vi "2_Trav_move.vi"(1 "Extra Command String":string, 3 "Home Z":T1, 5 "New Position":sgl[](array[numeric])=[0.0, 0.0, 0.0] format="%.2f", 9 "Backlash Compensation?":bool=TRUE, 11 "Simulate/Run":T2, 12 "Row Number":i32=-1, 13 "Currently on Point":i32=-1, 14 "Last Part of Move?":bool=TRUE) -> (4 "Trav Position achieved":sgl[](array[numeric]) format="%.2f", 6 "Error from Traverse named":string, 15 "Error String":string)   [LabVIEW 2022 SP3]
uses:
  Controls/User_Specific_mode.ctl
  Controls/Home.ctl
  Controls/Tunnel_Coordinates.ctl
  Globals/Extra_Commands_Global.vi
  Globals/Trav_pos_global.vi
  Globals/Constants_global.vi
panel:
  out "Offset (Tun Cord) 1-2":sgl[](array[numeric])
  out "Steps for 1st Traverse":sgl[][](array[numeric])
  out "File Content":string[](array[string])
  out "Traverse files":path[](array[path])
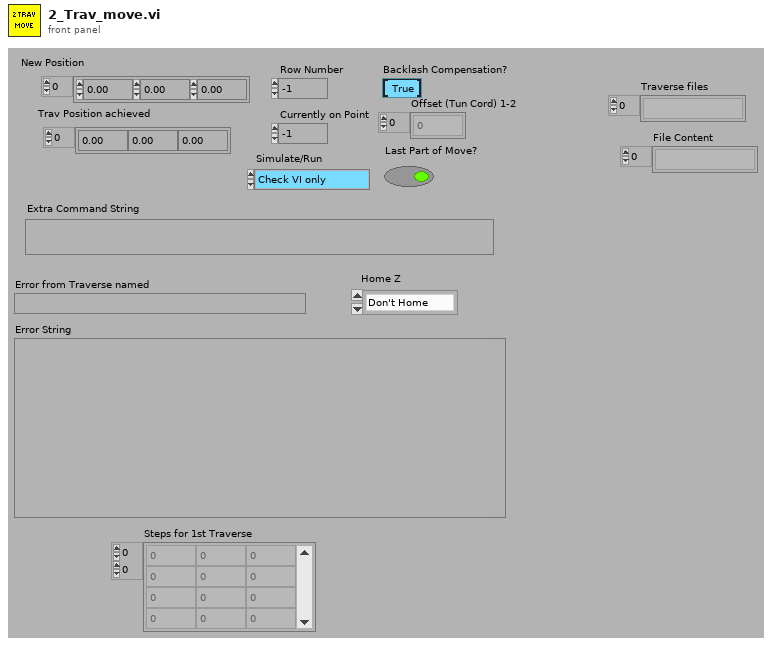
[diagram p1: front panel]
types:
  T1 = typedef "Home.ctl" = enum16{"Don't Home", "Home  +X", "Home  -X", "Home  +Y", "Home  -Y", "Home  +Z", "Home  -Z"}
  T2 = typedef "User_Specific_mode.ctl" = enum16{"Check VI only", "Run VI"}
  T3 = typedef "Tunnel_Coordinates.ctl" = enum16{"Work in Tunnel Coordinates", "Work in Model Coordinates"}
  T4 = enum16{"To Traverse Coordinates", "To User Coordinates"}
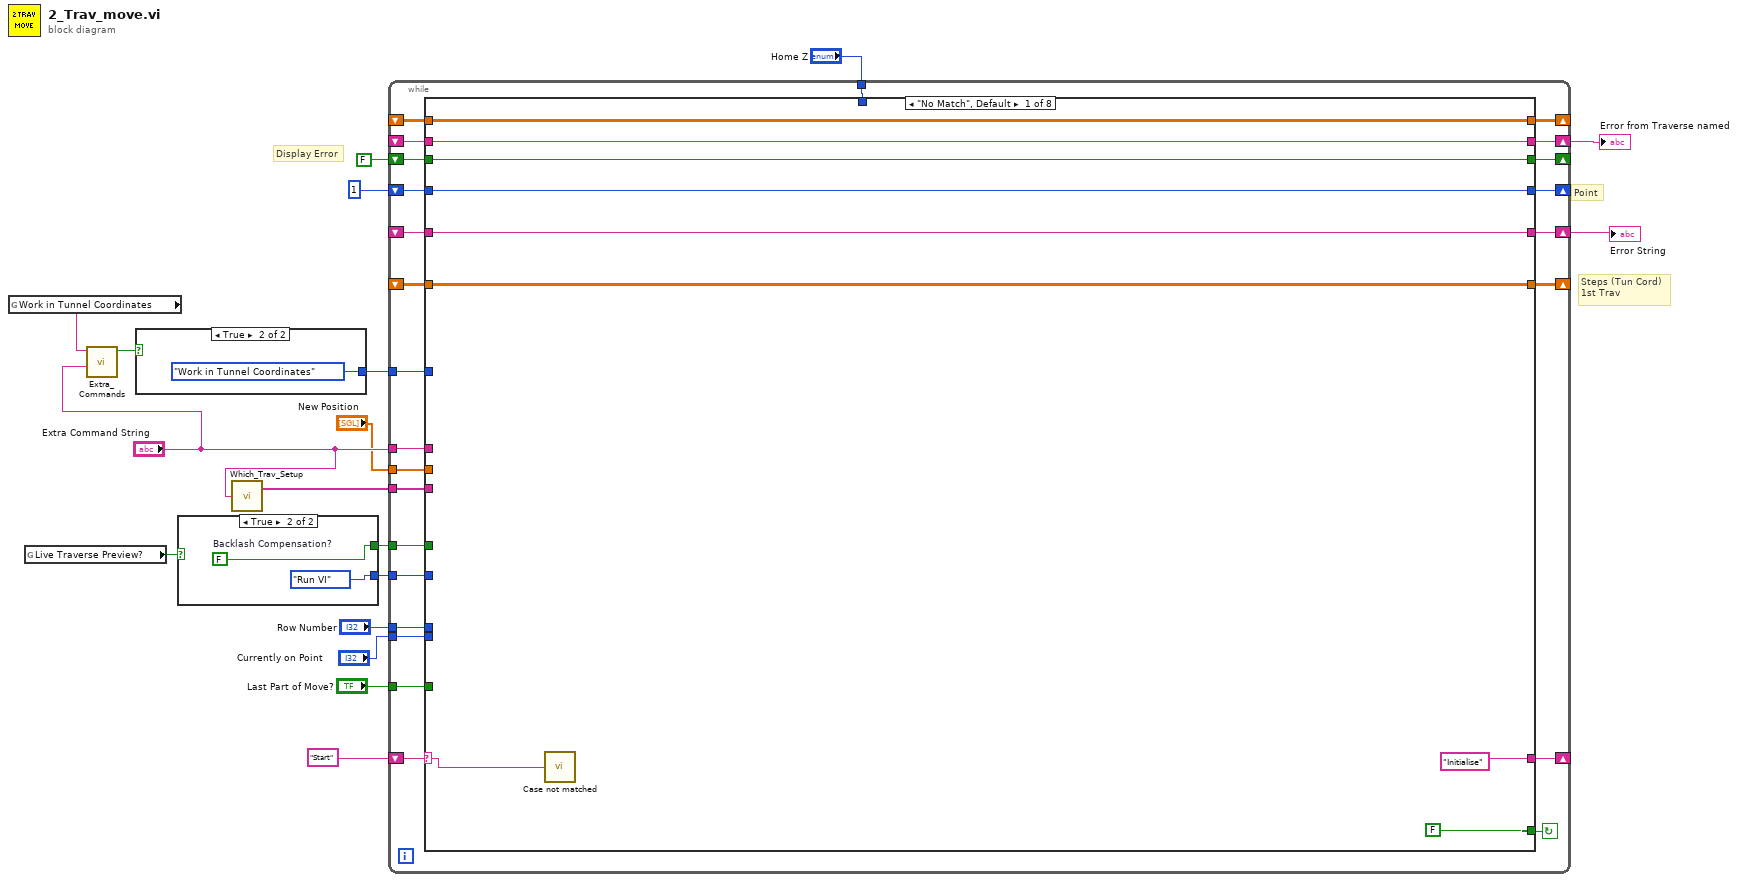
[diagram p0: block diagram]
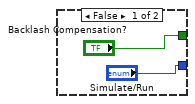
[diagram p2: hidden frame]
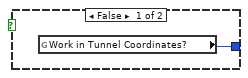
[diagram p3: hidden frame]
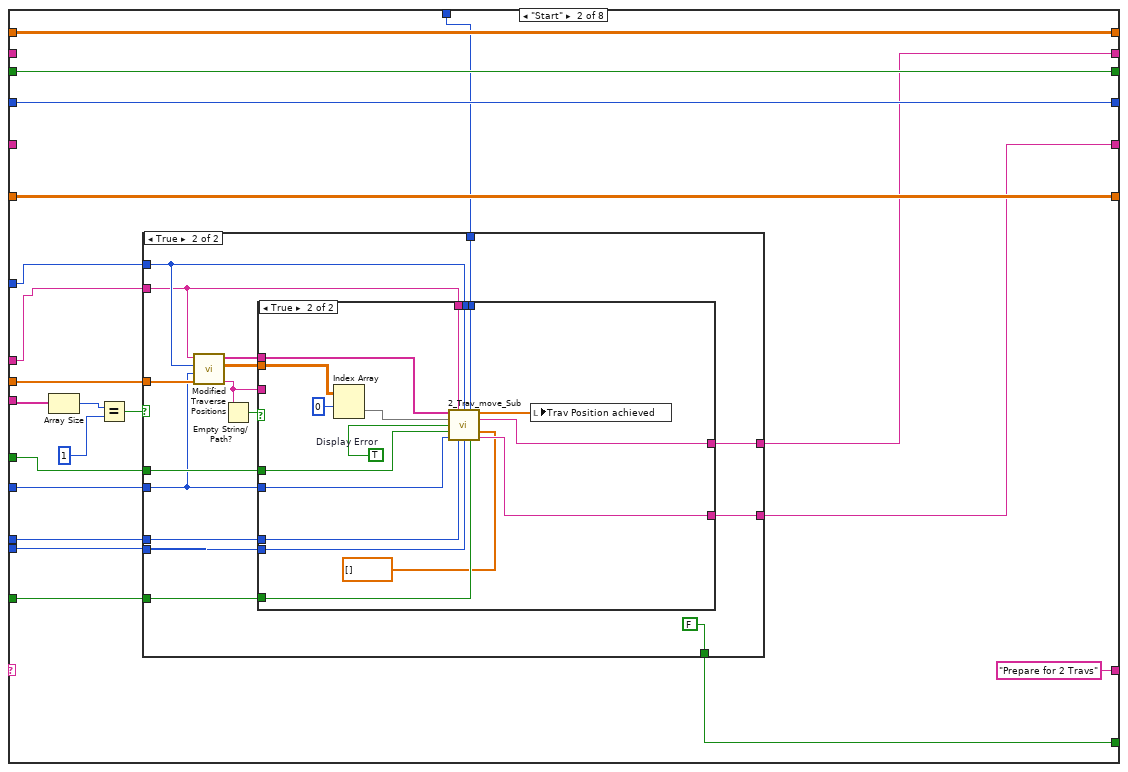
[diagram p4: hidden frame]
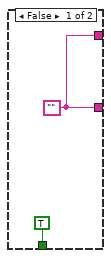
[diagram p5: hidden frame]
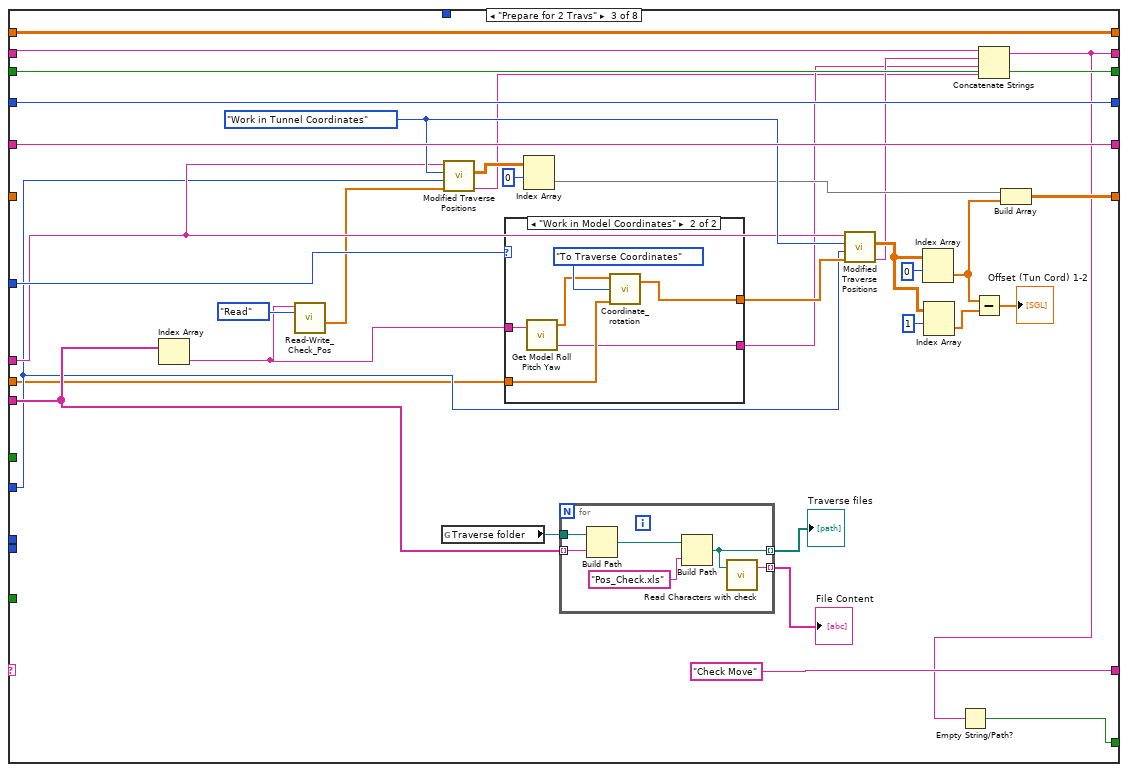
[diagram p7: hidden frame]
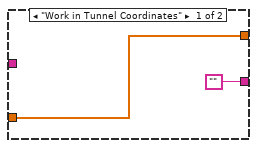
[diagram p8: hidden frame]
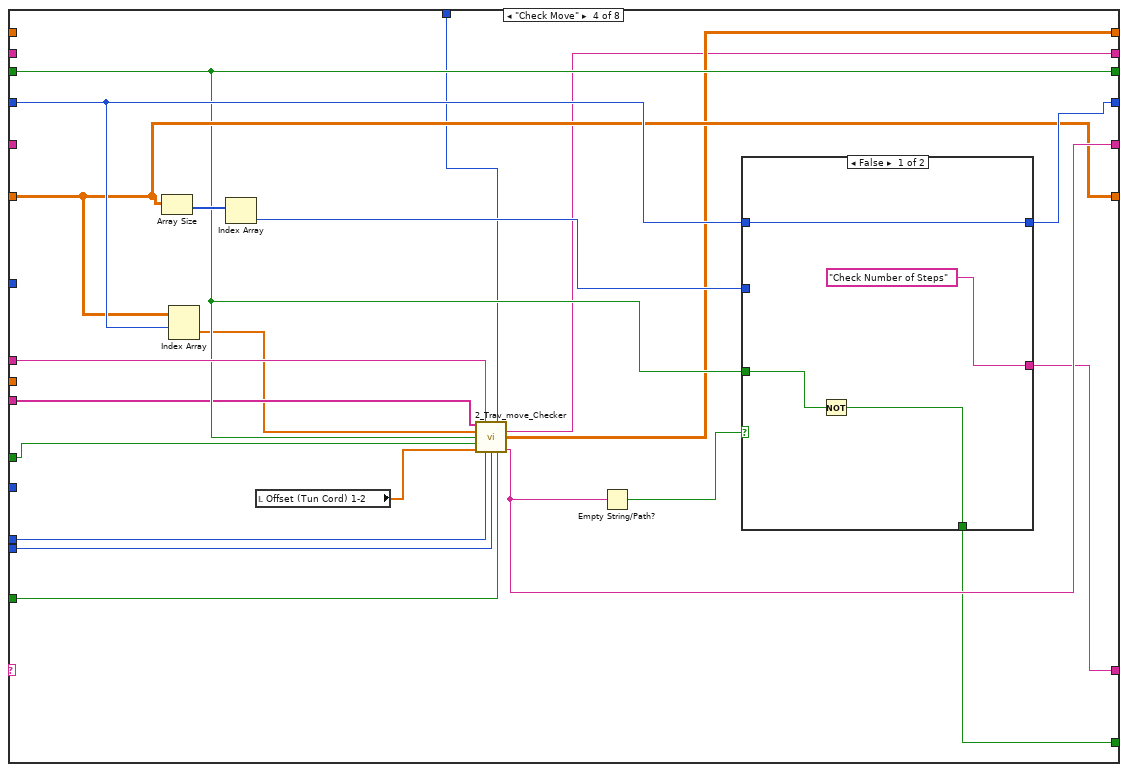
[diagram p9: hidden frame]
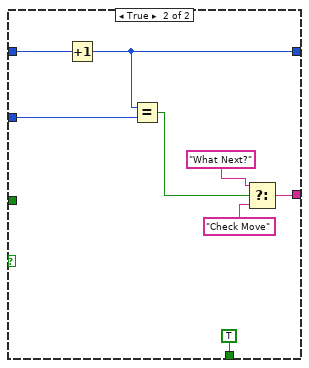
[diagram p10: hidden frame]
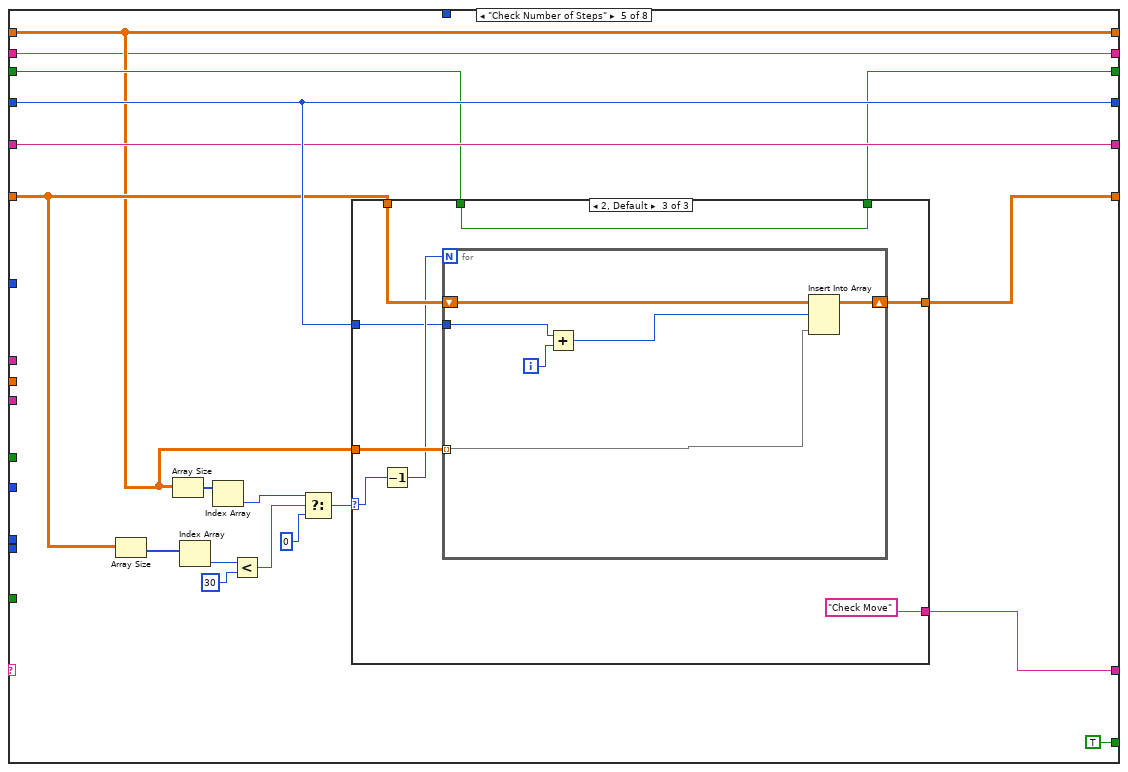
[diagram p11: hidden frame]
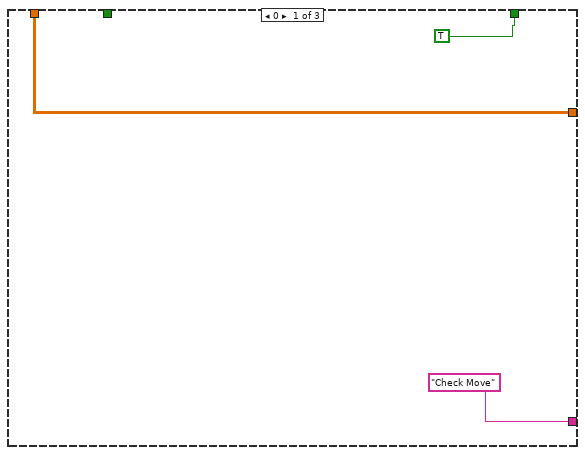
[diagram p12: hidden frame]
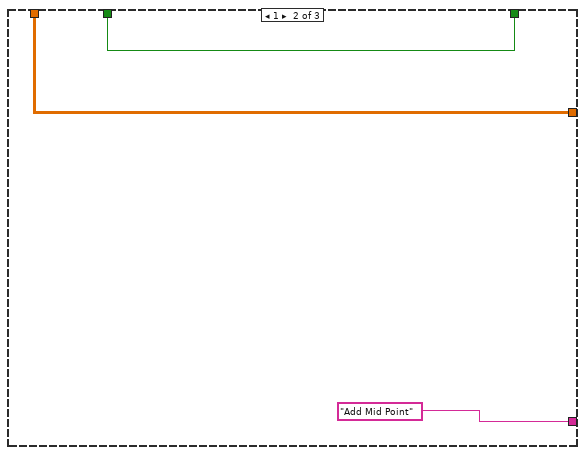
[diagram p13: hidden frame]
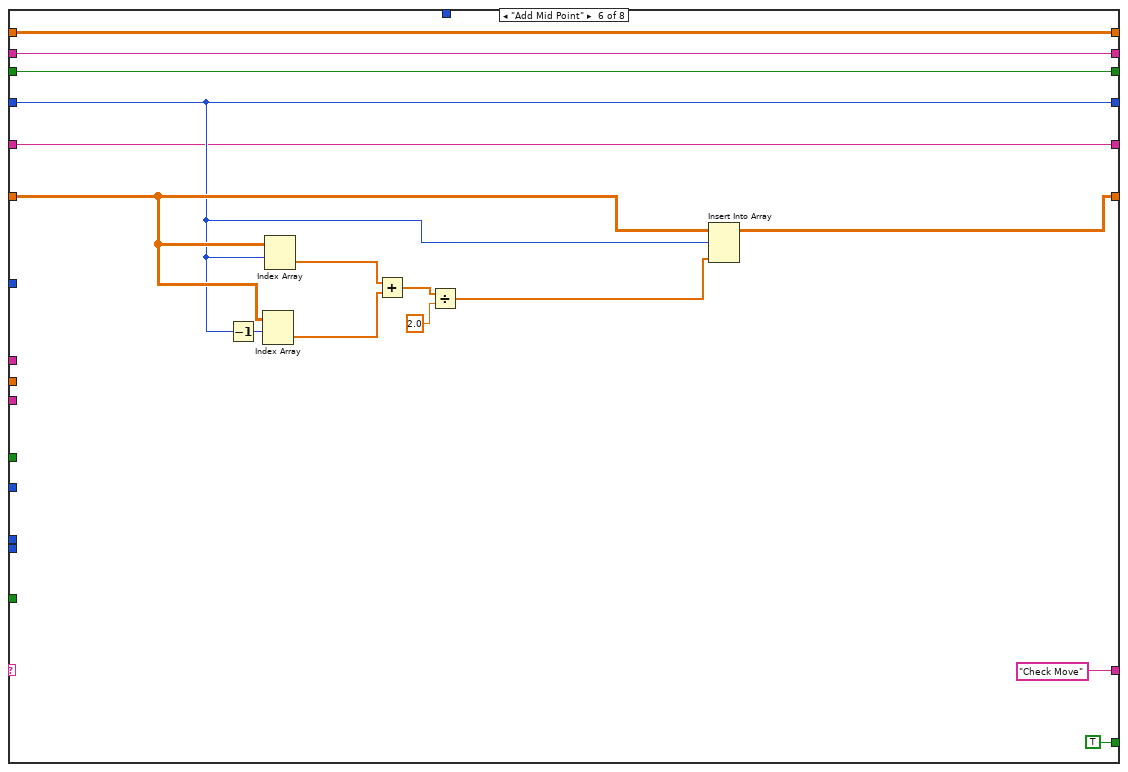
[diagram p14: hidden frame]
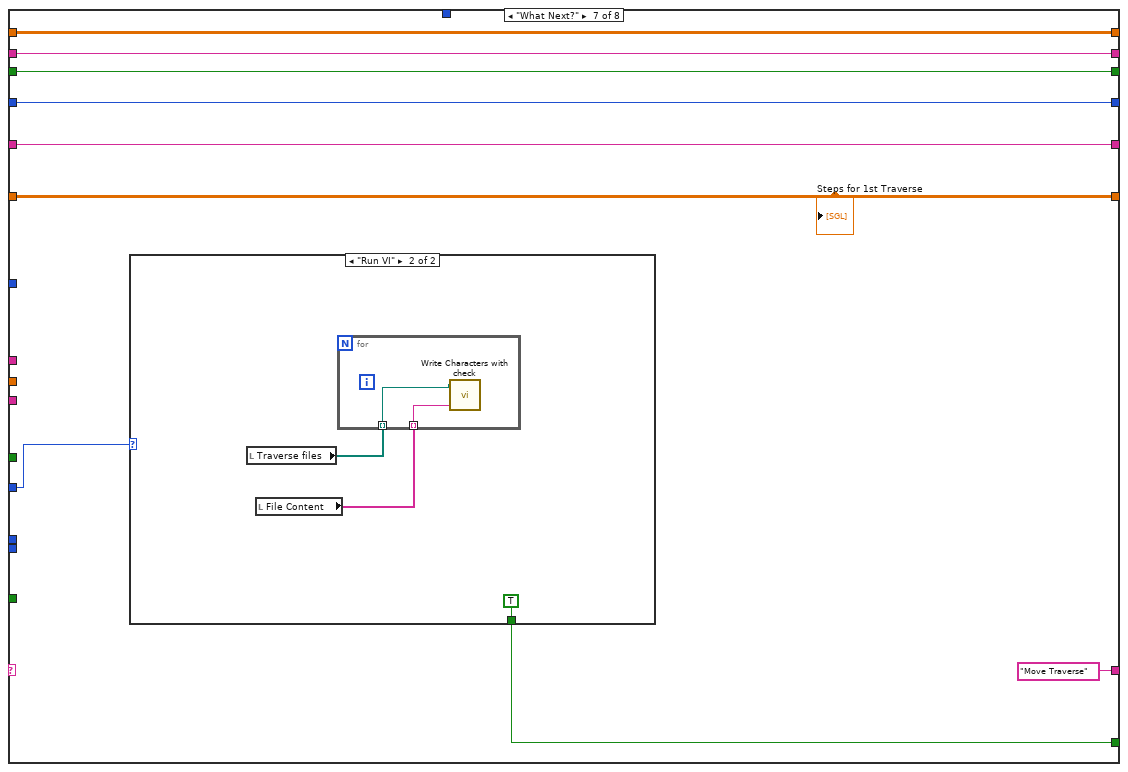
[diagram p15: hidden frame]
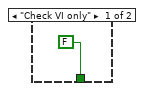
[diagram p16: hidden frame]
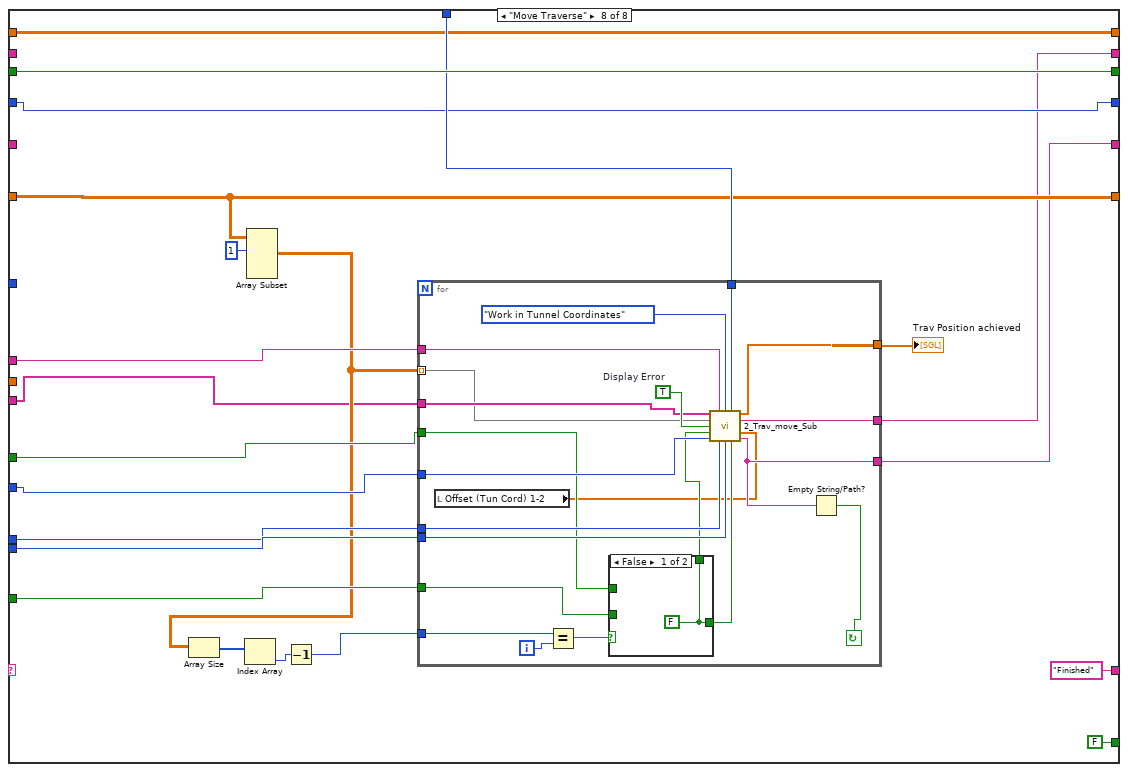
[diagram p17: hidden frame]
diagram:
  # "Steps (Tun Cord)\n1st Trav"
  # "Display Error"
  # "Point"
  n1 = global read "Extra_Commands_Global.vi" "Work in Tunnel Coordinates"() -> (w15:string)
  n2 = global read "Trav_pos_global.vi" "Live Traverse Preview?"() -> (w2:bool)
  n3 = call "Extra_Commands.vi"("String to Search"="Extra Command String", "Command"=w15) -> ("Command Found"=w16:bool)  [unwired: 1 in, 4 out]
  n4 = case shown="True" w16 {
    tunnel: [w19 Tunnel_Coordinates."Work in Tunnel Coordinates" ("Work in Tunnel Coordinates?")] -> w14
    frame False {
      n5 = global read "Trav_pos_global.vi" "Work in Tunnel Coordinates?"() -> (w19:T3)
    }
    frame True {
    }
  }
  n6 = case shown="True" w2 {
    tunnel: ["Backlash Compensation?" w23] -> w6
    tunnel: ["Simulate/Run" User_Specific_mode."Run VI" ("Simulate/Run")] -> w1
    frame False {
    }
    frame True {
      w23 = FALSE  # Backlash Compensation?
    }
  }
  n7 = call "Which_Trav_Setup.vi"("Extra Command String"="Extra Command String") -> ("Traverse Setups"=w12:string[])  [unwired: 2 out]
  n8 = while {
    shift-left: "Start" -> [w47]
    shift-right: [w48] -> _
    shift-right: [w40] -> _
    shift-left: _ -> [w46]
    tunnel: "Extra Command String" -> [w45]
    shift-right: [w44] -> w17
    shift-left: _ -> [w39]
    tunnel: w14 -> [w43]
    shift-right: [w41] -> _
    shift-left: 1 -> [w42]
    tunnel: w12 -> [w38]
    shift-right: [w36] -> _
    shift-left: FALSE -> [w37]
    shift-right: [w35] -> _
    shift-left: _ -> [w34]
    tunnel: "Home Z" -> [w33]
    tunnel: "Currently on Point" -> [w32]
    tunnel: "Row Number" -> [w31]
    tunnel: "Last Part of Move?" -> [w30]
    tunnel: w6 -> [w29]
    tunnel: w1 -> [w28]
    tunnel: "New Position" -> [w27]
    shift-right: [w26] -> w3
    shift-left: _ -> [w25]
    stop <- w49 continue-if-true
    n9 = case shown="\"No Match\", Default" w47 {
      selector: w47 -> [w50 _ _ _ _ _ _ _]
      tunnel: [FALSE w60 w116 w177 TRUE TRUE w251 FALSE] -> w49
      tunnel: ["Initialise" "Prepare for 2 Travs" "Check Move" w176 w213 "Check Move" "Move Traverse" "Finished"] -> w48
      tunnel: w46 -> [w56 w78 _ w175 w205 w244 w253 w280]
      tunnel: w45 -> [_ w65 w137 w184 _ _ _ w286]
      tunnel: [w55 w62 w146 w183 w210 w240 w257 w277] -> w44
      tunnel: w43 -> [_ w64 w142 _ _ _ _ _]
      tunnel: w42 -> [w54 w79 w147 w180 w211 w241 w258 w276]
      tunnel: [w54 w79 w147 w179 w211 w241 w258 w276] -> w41
      tunnel: [w56 w78 w141 w175 w212 w242 w253 w280] -> w40
      tunnel: w39 -> [w55 _ w146 _ w210 w240 w257 _]
      tunnel: w38 -> [_ w72 w143 w167 _ _ _ w266]
      tunnel: w37 -> [w53 w77 w148 w174 w208 w237 w255 w285]
      tunnel: [w53 w77 w148 w174 w209 w237 w255 w285] -> w36
      tunnel: [w52 w76 w149 w173 w198 w236 w254 w275] -> w35
      tunnel: w34 -> [w52 w76 w149 _ w198 w236 w254 w275]
      tunnel: w33 -> [_ w63 _ w172 _ _ _ w284]
      tunnel: w32 -> [_ w67 _ w171 _ _ _ w283]
      tunnel: w31 -> [_ w68 _ w170 _ _ _ w282]
      tunnel: w30 -> [_ w66 _ w169 _ _ _ w281]
      tunnel: w29 -> [_ w70 _ w168 _ _ _ w271]
      tunnel: w28 -> [_ w69 w136 _ _ _ w252 w272]
      tunnel: w27 -> [_ w71 w125 _ _ _ _ _]
      tunnel: [w51 w59 w117 w164 w197 w235 w250 w265] -> w26
      tunnel: w25 -> [w51 _ w121 _ w197 w235 w250 _]
      frame "No Match", Default {
        n10 = call "Case not matched.vi"("Case Name not Matched"=w50) -> ()
      }
      frame "Start" {
        n11 = Array Size(array=w72) -> (size(s)=w75:i32)
        n12 = Equal?(x=w75, y=1) -> (x = y?=w73:bool)
        n13 = case shown="True" w73 {
          tunnel: w71 -> [_ w89]
          tunnel: w70 -> [_ w97]
          tunnel: w69 -> [_ w88]
          tunnel: w68 -> [_ w96]
          tunnel: w67 -> [_ w95]
          tunnel: w66 -> [_ w94]
          tunnel: w65 -> [_ w86]
          tunnel: w64 -> [_ w87]
          tunnel: w63 -> [_ w93]
          tunnel: [w80 w92] -> w62
          tunnel: [TRUE FALSE] -> w60
          tunnel: [w80 w84] -> w59
          frame False {
            w80 = ""
          }
          frame True {
            n14 = call "Modified Traverse Positions.vi"("Input Position"=w89, "Simulate/Run"=w88, "Work in Tunnel Coordinates?"=w87, "Extra Command String"=w86) -> ("Error String"=w82:string, "Traverse Positions"=w85:sgl[][], "Traverse Setups"=w90:string[])  [unwired: 1 out]
            n15 = Empty String/Path?(string/path=w82) -> (empty?=w83:bool)
            n16 = case shown="True" w83 {
              tunnel: w97 -> [_ w114]
              tunnel: w96 -> [_ w113]
              tunnel: w95 -> [_ w112]
              tunnel: w94 -> [_ w111]
              tunnel: w93 -> [_ w110]
              tunnel: [w98 w108] -> w92
              tunnel: w90 -> [_ w106]
              tunnel: w88 -> [_ w105]
              tunnel: w87 -> [_ w104]
              tunnel: w86 -> [_ w103]
              tunnel: w85 -> [_ w102]
              tunnel: [w98 w99] -> w84
              tunnel: w82 -> [w98 _]
              frame False {
              }
              frame True {
                w115 = TRUE  # Display Error
                n17 = Index Array(array=w102, index (row)=0) -> (element=w100:sgl[])  [unwired: 1 in]
                n18 = call "2_Trav_move_Sub.vi"("Traverse Setups"=w106, "Extra Command String"=w103, "Work in Tunnel Coordinates?"=w104, "Home Z"=w110, "Traverse Positions"=w100, "Display Error"=w115, "Backlash Compensation?"=w114, "Offset (Tun Cord) 1-2"=sgl[] [], "Simulate/Run"=w105, "Row Number"=w113, "Currently on Point"=w112, "Last Part of Move?"=w111) -> ("Trav Position achieved"=w109:sgl[], "Error from Traverse named"=w99:string, "Error String"=w108:string)  [unwired: 1 in]
                n19 = local write "Trav Position achieved"(w109) -> ()
              }
            }
          }
        }
      }
      frame "Prepare for 2 Travs" {
        w139 = Tunnel_Coordinates."Work in Tunnel Coordinates" ("Work in Tunnel Coordinates?")
        n20 = Index Array(array=w143) -> (element=w138:string)  [unwired: 1 in]
        n21 = call "Read-Write_Check_Pos.vi"("Mode"=enum16{"Read", "Write"}."Read", "Traverse Name"=w138) -> ("Position Output"=w126:sgl[])  [unwired: 5 in, 2 out]
        n22 = global read "Constants_global.vi" "Traverse folder"() -> (w124:path)
        n23 = call "Modified Traverse Positions.vi"("Input Position"=w126, "Simulate/Run"=w136, "Work in Tunnel Coordinates?"=w139, "Extra Command String"=w137) -> ("Error String"=w118:string, "Traverse Positions"=w135:sgl[][])  [unwired: 2 out]
        n24 = case shown="\"Work in Model Coordinates\"" w142 {
          tunnel: w125 -> [w157 w162]
          tunnel: [w157 w161] -> w140
          tunnel: w138 -> [_ w160]
          tunnel: ["" w158] -> w119
          frame "Work in Tunnel Coordinates" {
          }
          frame "Work in Model Coordinates" {
            n25 = call "Get Model Roll Pitch Yaw.vi"("Traverse Name"=w160) -> ("Model:    Roll        Pitch         Yaw  (deg)"=w159:sgl[], "Error String"=w158:string)  [unwired: 1 in, 1 out]
            n26 = call "Coordinate_rotation.vi"("Roll-Pitch-Yaw"=w159, "Input Position"=w162, "Mode"=T4."To Traverse Coordinates") -> ("Output Position"=w161:sgl[])  [unwired: 2 in, 1 out]
          }
        }
        n27 = Index Array(array=w135, index (row)=0) -> (element=w133:sgl[])  [unwired: 1 in]
        n28 = for {
          tunnel: w124 -> [w153]
          tunnel: w143 -> [w152] mode=indexing
          tunnel: [w150] -> w122 mode=indexing
          tunnel: [w151] -> w123 mode=indexing
          n29 = Build Path(base path=w153, name or relative path=w152) -> (appended path=w154:path)
          n30 = Build Path(base path=w154, name or relative path="Pos_Check.xls" ("string")) -> (appended path=w151:path)
          n31 = call "Read Characters with check.vi"("file (use dialog)"=w151) -> ("Read String"=w150:string)  [unwired: 1 in, 1 out]
        }
        "Traverse files" <- w123
        "File Content" <- w122
        n32 = call "Modified Traverse Positions.vi"("Input Position"=w140, "Simulate/Run"=w136, "Work in Tunnel Coordinates?"=w139, "Extra Command String"=w137) -> ("Error String"=w120:string, "Traverse Positions"=w130:sgl[][])  [unwired: 2 out]
        n33 = Index Array(array=w130, index (row)=0) -> (element=w129:sgl[])  [unwired: 1 in]
        n34 = Index Array(array=w130, index (row)=1) -> (element=w128:sgl[])  [unwired: 1 in]
        n35 = Subtract(x=w129, y=w128) -> (x-y=→"Offset (Tun Cord) 1-2":sgl[])
        n36 = Concatenate Strings(w121, w120, w119, w118) -> (w117:string)
        n37 = Empty String/Path?(string/path=w117) -> (empty?=w116:bool)
        n38 = Build Array(w133, w129) -> (w141:sgl[][])
      }
      frame "Check Move" {
        n39 = Array Size(array=w175) -> (size(s)=w182:i32[])
        n40 = Index Array(array=w175, index (row)=w180) -> (element=w166:sgl[])  [unwired: 1 in]
        n41 = Index Array(array=w182) -> (element=w178:i32)  [unwired: 1 in]
        n42 = local read "Offset (Tun Cord) 1-2"() -> (w165:sgl[])
        n43 = call "2_Trav_move_Checker.vi"("Traverse Setups"=w167, "Extra Command String"=w184, "Home Z"=w172, "Traverse Positions (Tun Cord)"=w166, "Display Error"=w174, "Backlash Compensation?"=w168, "Offset (Tun Cord) 1-2"=w165, "Row Number"=w170, "Currently on Point"=w171, "Last Part of Move?"=w169) -> ("Error from Traverse named"=w164:string, "Steps  for First Trav"=w173:sgl[][], "Error String"=w183:string)  [unwired: 2 in, 1 out]
        n44 = Empty String/Path?(string/path=w183) -> (empty?=w181:bool)
        n45 = case shown="False" w181 {
          tunnel: w180 -> [w187 w196]
          tunnel: [w187 w195] -> w179
          tunnel: w178 -> [_ w194]
          tunnel: [w185 TRUE] -> w177
          tunnel: ["Check Number of Steps" w189] -> w176
          tunnel: w174 -> [w186 _]
          frame False {
            n46 = Not(x=w186) -> (.not. x?=w185:bool)
          }
          frame True {
            n47 = Increment(x=w196) -> (x+1=w195:i32)
            n48 = Equal?(x=w195, y=w194) -> (x = y?=w192:bool)
            n49 = Select(t="What Next?", s=w192, f="Check Move") -> (s? t:f=w189:string)
          }
        }
      }
      frame "Check Number of Steps" {
        n50 = Array Size(array=w205) -> (size(s)=w206:i32[])
        n51 = Array Size(array=w198) -> (size(s)=w214:i32[])
        n52 = Index Array(array=w206) -> (element=w203:i32)  [unwired: 1 in]
        n53 = Index Array(array=w214) -> (element=w200:i32)  [unwired: 1 in]
        n54 = Less?(x=w203, y=30) -> (x < y?=w201:bool)
        n55 = Select(t=w200, s=w201, f=0) -> (s? t:f=w204:i32)
        n56 = case shown="2, Default" w204 {
          selector: w204 -> [_ _ w226]
          tunnel: ["Check Move" "Add Mid Point" "Check Move"] -> w213
          tunnel: w211 -> [_ _ w224]
          tunnel: w198 -> [_ _ w228]
          tunnel: w205 -> [w217 w219 w227]
          tunnel: [w217 w219 w223] -> w212
          tunnel: [TRUE w218 w221] -> w209
          tunnel: w208 -> [_ w218 w221]
          frame 0 {
          }
          frame 1 {
          }
          frame 2, Default {
            n57 = Decrement(x=w226) -> (x-1=w225:i32)
            n58 = for {
              N: w225 -> [_]
              tunnel: w228 -> [w230] mode=indexing
              shift-right: [w229] -> w223
              shift-left: w227 -> [w231]
              tunnel: w224 -> [w233]
              i -> [w234]
              n59 = Add(x=w233, y=w234) -> (x+y=w232:i32)
              n60 = Insert Into Array(array=w231, index (row)=w232, new element=w230) -> (w229:sgl[][])  [unwired: 1 in]
            }
          }
        }
      }
      frame "Add Mid Point" {
        n61 = Decrement(x=w241) -> (x-1=w249:i32)
        n62 = Index Array(array=w244, index (row)=w249) -> (element=w247:sgl[])  [unwired: 1 in]
        n63 = Index Array(array=w244, index (row)=w241) -> (element=w248:sgl[])  [unwired: 1 in]
        n64 = Add(x=w248, y=w247) -> (x+y=w246:sgl[])
        n65 = Divide(x=w246, y=sgl 2.0) -> (x/y=w243:sgl[])
        n66 = Insert Into Array(array=w244, index (row)=w241, new element=w243) -> (w242:sgl[][])  [unwired: 1 in]
      }
      frame "What Next?" {
        n67 = case shown="\"Run VI\"" w252 {
          tunnel: [FALSE TRUE] -> w251
          frame "Check VI only" {
          }
          frame "Run VI" {
            n68 = local read "Traverse files"() -> (w261:path[])
            n69 = local read "File Content"() -> (w260:string[])
            n70 = for {
              tunnel: w260 -> [w263] mode=indexing
              tunnel: w261 -> [w264] mode=indexing
              n71 = call "Write Characters with check.vi"("String to Write"=w263, "file (use dialog)"=w264) -> ()  [unwired: 2 in, 1 out]
            }
          }
        }
        "Steps for 1st Traverse" <- w253
      }
      frame "Move Traverse" {
        n72 = Array Subset(array=w280, index (row)=1 ("index")) -> (w269:sgl[][])  [unwired: 3 in]
        n73 = Array Size(array=w269) -> (size(s)=w270:i32[])
        n74 = Index Array(array=w270) -> (element=w268:i32)  [unwired: 1 in]
        n75 = Decrement(x=w268) -> (x-1=w267:i32)
        n76 = for {
          tunnel: w269 -> [w288] mode=indexing
          tunnel: w286 -> [w299]
          tunnel: w284 -> [w307]
          tunnel: w283 -> [w306]
          tunnel: w282 -> [w305]
          tunnel: w281 -> [w293]
          tunnel: w271 -> [w291]
          tunnel: [w304] -> w278
          tunnel: [w303] -> w265
          tunnel: [w301] -> w277
          tunnel: w272 -> [w298]
          tunnel: w267 -> [w296]
          tunnel: w266 -> [w290]
          i -> [w297]
          stop <- w302 continue-if-true
          w300 = TRUE  # Display Error
          n77 = local read "Offset (Tun Cord) 1-2"() -> (w287:sgl[])
          n78 = Equal?(x=w296, y=w297) -> (x = y?=w295:bool)
          n79 = case shown="False" w295 {
            tunnel: [w308 w310] -> w294
            tunnel: w293 -> [_ w310]
            tunnel: [w308 w309] -> w292
            tunnel: w291 -> [_ w309]
            frame False {
              w308 = FALSE
            }
            frame True {
            }
          }
          n80 = call "2_Trav_move_Sub.vi"("Traverse Setups"=w290, "Extra Command String"=w299, "Work in Tunnel Coordinates?"=Tunnel_Coordinates."Work in Tunnel Coordinates", "Home Z"=w307, "Traverse Positions"=w288, "Display Error"=w300, "Backlash Compensation?"=w292, "Offset (Tun Cord) 1-2"=w287, "Simulate/Run"=w298, "Row Number"=w305, "Currently on Point"=w306, "Last Part of Move?"=w294) -> ("Trav Position achieved"=w304:sgl[], "Error from Traverse named"=w303:string, "Error String"=w301:string)  [unwired: 1 in]
          n81 = Empty String/Path?(string/path=w301) -> (empty?=w302:bool)
        }
        "Trav Position achieved" <- w278
      }
    }
  }
  "Error String" <- w17
  "Error from Traverse named" <- w3
